vi "Initialize HD44780.vi"(6 "font configuration (5x8 & 2 lines)":T2(ring), 8 "error in (no error)":errorcluster, 9 "screen size":T1(ring)=enum."16x2", 10 "device index":i8, 11 "FPGA VI Reference in":refnum<k20>) -> (0 "error out":errorcluster, 3 "LCD out":refnum<class "Character LCD.lvclass">)   [LabVIEW 2017, in "HD44780 Host.lvlib"]
doc: "ORIGINAL CODE: \nBy: National Instruments\n NI LabVIEW RIO Evaluation Kit\n Code example \"5- Startup Application\"\n www.ni.com/embeddedsystems\n\nUPDATED CODE: Adds NI SystemLink and NI AWS LabVIEW Tookit functionality for demonstration. \nBy: James Tillett\n Endeavor Engineering Inc.\n www.endeavoreng.com"
uses:
  HD44780 Host.lvlib
  Internal/LCD Class/Character LCD.lvclass
  Internal/HD44780/HD44780.lvclass
  E:/Working/SystemLink Demo NIWeek 2017_Tillett/sbRIO Eval SystemLink Demo/LabVIEW/Real-Time/EmbeddedDisplay/Hitachi HD44780/Host/Internal/LCD Class/Character LCD.lvclass
  Common/HD44780 Common.lvlib
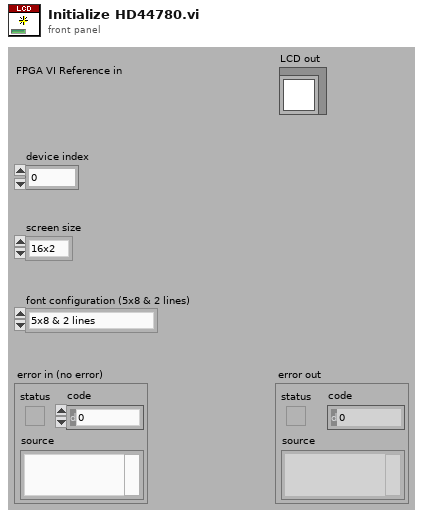
[diagram p1: front panel]
types:
  T1 = enum8{"8x1", "8x2", "12x4", "16x1", "16x2", "16x4", "20x1", "20x2", "20x4", "24x1", "24x2", "40x2", "40x4"}
  T2 = enum8{"5x8 & 2 lines", "5x10 & 1 line", "5x8 & 1 line"}
  T3 = cluster{"FPGA VI Reference":refnum<k20>, "device index":i8, "screen size":enum8{"8x1", "8x2", "12x4", "16x1", "16x2", "16x4", "20x1", "20x2", "20x4", "24x1", "24x2", "40x2", "40x4"}, "font size":enum8{"5x8", "5x10"}, "auto wrap":bool, "alignment":enum16{"None", "Left", "Center", "Right"}, "number of line":enum8{"1 line", "2 lines"}, "shift 0":i8, "entry mode 0":enum8{"increment & no shift", "increment & shift", "decrement & no shift", "decrement & shift"}, "shift 1":i8, "entry mode 1":enum8{"increment & no shift", "increment & shift", "decrement & no shift", "decrement & shift"}}
  T4 = enum8{"increment & no shift", "increment & shift", "decrement & no shift", "decrement & shift"}
  T5 = enum8{"cursor off", "cursor on & no blink", "cursor on & blink"}
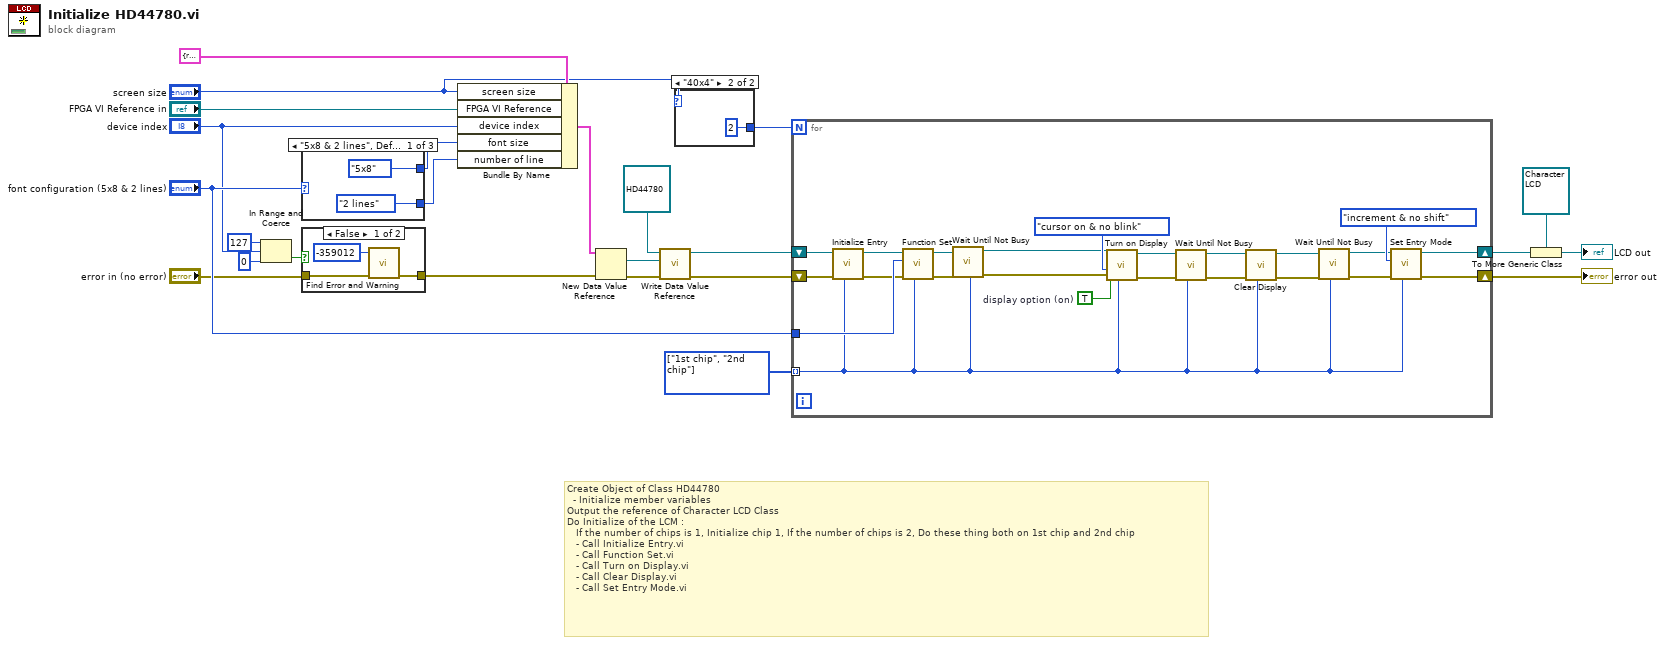
[diagram p0: block diagram]
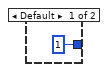
[diagram p3: hidden frame]
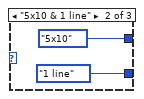
[diagram p4: hidden frame]
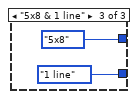
[diagram p5: hidden frame]
diagram:
  w21 = enum16{"1st chip", "2nd chip"}[] [enum."1st chip", enum."2nd chip"] items=["1st chip", "2nd chip"] ("initialized array")
  # "Create Object of Class HD44780\n  - Initialize member variables\nOutput the reference of Character LCD Class \nDo Initialize of the LCM :\n   If the number of chips is 1, Initialize chip 1, If the number of chips is 2, Do these thing both on 1st chip and 2nd chip \n   - Call Initialize Entry.vi \n   - Call Function Set.vi\n   - Call Turn on Display.vi\n   - Call Clear Display.vi\n   - Call Set Entry Mode.vi"
  n1 = In Range and Coerce(upper limit=i8 127, x="device index", lower limit=i8 0) -> (In Range?=w5:bool)  [unwired: 1 out]
  n2 = case shown="\"5x8 & 2 lines\", Default" "font configuration (5x8 & 2 lines)" {
    tunnel: [enum8{"5x8", "5x10"}."5x8" ("font size") enum8{"5x8", "5x10"}."5x10" ("font size") enum8{"5x8", "5x10"}."5x8" ("font size")] -> w20
    tunnel: [enum8{"1 line", "2 lines"}."2 lines" ("line number") enum8{"1 line", "2 lines"}."1 line" ("line number") enum8{"1 line", "2 lines"}."1 line" ("line number")] -> w19
    frame "5x8 & 2 lines", Default {
    }
    frame "5x10 & 1 line" {
    }
    frame "5x8 & 1 line" {
    }
  }
  n3 = case shown="False" w5 {
    tunnel: [w32 w34] -> w3
    tunnel: "error in (no error)" -> [w31 w34]
    frame False {
      n4 = call "Find Error and Warning.vi"("error in (no error)"=w31, "error code"=-359012) -> ("error out"=w32:errorcluster)  [unwired: 9 in]
    }
    frame True {
    }
  }
  n5 = Bundle By Name(cluster=T3 {"FPGA VI Reference"=refnum, "device index"=0, "screen size"=enum."8x1", "font size"=enum."5x8", "auto wrap"=FALSE, "alignment"=enum."None", "number of line"=enum."1 line", "shift 0"=0, "entry mode 0"=enum."increment & no shift", "shift 1"=0, "entry mode 1"=enum."increment & no shift"} ("Cluster of class private data"), "screen size"="screen size", "FPGA VI Reference"="FPGA VI Reference in", "device index"="device index", "font size"=w20, "number of line"=w19) -> (w14:T3)
  n6 = New Data Value Reference(data value=w14, error in=w3) -> (data value reference=w9:refnum<data-value>, error out=w18:errorcluster)
  n7 = call "Write Data Value Reference.vi"("error in (no error)"=w18, "data value reference"=w9, "HD44780 in"=refnum<class "HD44780.lvclass"> refnum ("HD44780.lvclass")) -> ("error out"=w17:errorcluster, "HD44780 out"=w16:refnum<class "HD44780.lvclass">)  [unwired: 7 in]
  n8 = case shown="\"40x4\"" "screen size" {
    tunnel: [1 2] -> w22
    frame Default {
    }
    frame "40x4" {
    }
  }
  n9 = for {
    N: w22 -> [_]
    tunnel: "font configuration (5x8 & 2 lines)" -> [w59]
    tunnel: w21 -> [w39] mode=indexing
    shift-right: [w58] -> w23
    shift-left: w17 -> [w57]
    shift-right: [w50] -> w10
    shift-left: w16 -> [w56]
    w53 = TRUE  # display option (on)
    n10 = call "Initialize Entry.vi"("chip select (1st chip)"=w39, "error in (no error)"=w57, "HD44780 in"=w56) -> ("error out"=w54:errorcluster, "HD44780 out"=w55:refnum<class "HD44780.lvclass">)  [unwired: 7 in]
    n11 = call "Function Set.vi"("chip select (1st chip)"=w39, "error in (no error)"=w54, "font configuration (5x8 & 2 lines)"=w59, "HD44780 in"=w55) -> ("error out"=w49:errorcluster, "HD44780 out"=w47:refnum<class "HD44780.lvclass">)  [unwired: 6 in]
    n12 = call "Wait Until Not Busy.vi"("chip select (1st chip)"=w39, "error in"=w49, "HD44780 in"=w47) -> ("error out"=w48:errorcluster, "HD44780 out"=w46:refnum<class "HD44780.lvclass">)  [unwired: 7 in]
    n13 = call-dynamic "Turn on Display.vi"("chip select  (1st chip)"=w39, "error in (no error)"=w48, "cursor option"=T5."cursor on & no blink" ("cursor option (on & no blink)"), "display on?"=w53, "HD44780 in"=w46) -> ("error out"=w44:errorcluster, "HD44780 out"=w45:refnum<class "HD44780.lvclass">)  [unwired: 5 in]
    n14 = call "Wait Until Not Busy.vi"("chip select (1st chip)"=w39, "error in"=w44, "HD44780 in"=w45) -> ("error out"=w42:errorcluster, "HD44780 out"=w43:refnum<class "HD44780.lvclass">)  [unwired: 7 in]
    n15 = call-dynamic "Clear Display.vi"("chip select  (1st chip)"=w39, "error in (no error)"=w42, "HD44780 in"=w43) -> ("error out"=w40:errorcluster, "HD44780 out"=w41:refnum<class "HD44780.lvclass">)  [unwired: 7 in]
    n16 = call "Wait Until Not Busy.vi"("chip select (1st chip)"=w39, "error in"=w40, "HD44780 in"=w41) -> ("error out"=w37:errorcluster, "HD44780 out"=w38:refnum<class "HD44780.lvclass">)  [unwired: 7 in]
    n17 = call-dynamic "Set Entry Mode.vi"("chip select  (1st chip)"=w39, "error in (no error)"=w37, "entry mode"=T4."increment & no shift", "HD44780 in"=w38) -> ("error out"=w58:errorcluster, "HD44780 out"=w50:refnum<class "HD44780.lvclass">)  [unwired: 6 in]
  }
  "error out" <- w23
  n18 = To More Generic Class(target class=refnum<class "Character LCD.lvclass"> refnum ("Character LCD.lvclass"), reference=w10) -> (generic class reference=→"LCD out":refnum<class "Character LCD.lvclass">)
